vi "make_gasid_unit_ring.vi"() -> ()   [LabVIEW 2013]
uses:
  <vilib>/Utility/file.llb/Read From Spreadsheet File (string).vi
panel:
  in  "uom1":T1(ring)
  in  "gid2":T2(ring)
  out "Duplicates":string[](array[string])
  out "Uniques":string[](array[string])
  out "all rows":string[][](array[string])
  in  "Ring":u16(ring) items=["ERR", "SCCM", "SLM", "%", "V", "MV", "CNT", "NLM", "SLS", "NLS", "SLH", "NLH", "SMLM", "NMLM", "SMLS", "NMLS", "SMLH", "NMLH", "NCCM", "SCCS", "NCCS", "SCCH", "NCCH", "SCFM", "NCFM", "SCFS", "NCFS", "SCFH", "NCFH", "SCMM", "NCMM", "SCMS", "NCMS", "SCMH", "NCMH", "SCIM", "NCIM", "SCIS", "NCIS", "SCIH", "NCIH", "LBM", "LBS", "LBH", "KgM", "KgS", "KgH", "GRM", "GMS", "GRH", "MolM", "MolS", "MolH", "KMolM", "KMolS", "KMolH", "W", "BPS", "Sec", "Min", "Hrs", "WH", "Torr", "Bar", "Pa", "inH2O", "PSIA", "PSIG"]
  in  "file path (dialog if empty)":path
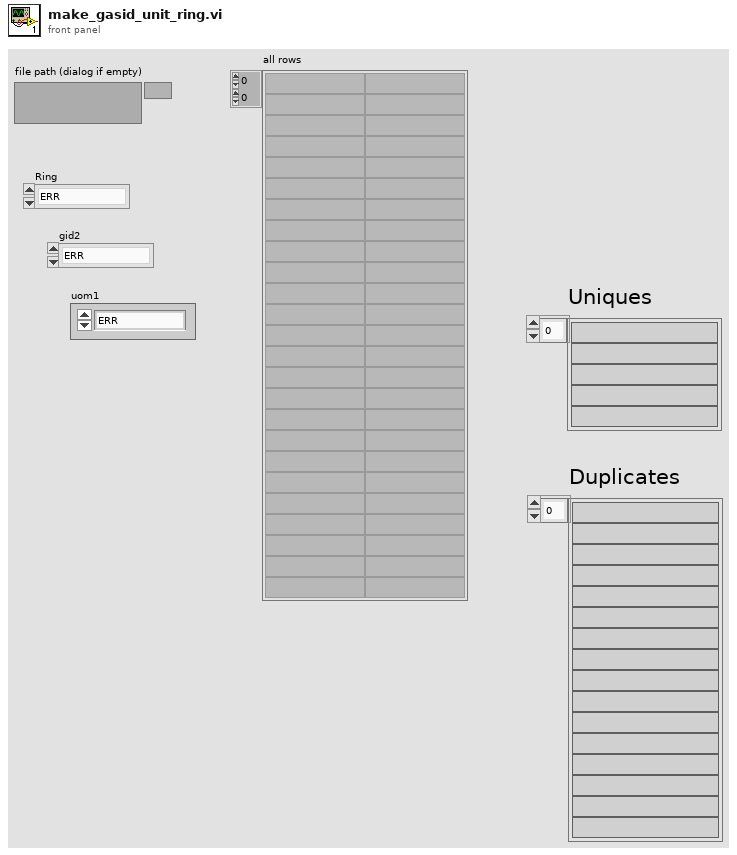
[diagram p1: front panel]
types:
  T1 = enum16{"ERR", "SCCM", "SLM", "%", "V", "MV", "CNT", "NLM", "SLS", "NLS", "SLH", "NLH", "SMLM", "NMLM", "SMLS", "NMLS", "SMLH", "NMLH", "NCCM", "SCCS", "NCCS", "SCCH", "NCCH", "SCFM", "NCFM", "SCFS", "NCFS", "SCFH", "NCFH", "SCMM", "NCMM", "SCMS", "NCMS", "SCMH", "NCMH", "SCIM", "NCIM", "SCIS", "NCIS", "SCIH", "NCIH", "LBM", "LBS", "LBH", "KgM", "KgS", "KgH", "GRM", "GMS", "GRH", "MolM", "MolS", "MolH", "KMolM", "KMolS", "KMolH", "W", "BPS", "Sec", "Min", "Hrs", "WH", "Torr", "Bar", "Pa", "inH2O", "PSIA", "PSIG"}
  T2 = enum16{"ERR", "1", "2", "C3H6O_1", "C2H3N", "C2H2", "Air", "C3H4_1", "NH3", "Ar", "AsH3", "C6H6", "BCl3", "BF3", "Br2", "15", "16", "CBrF3", "C4H10_1", "19", "C4H8_1", "CO2", "CS2", "CO", "CCl4", "COS", "Cl2", "ClF3", "28", "29", "CHCl3", "31", "32", "C4H8_2", "C2N2", "ClCN", "C4H8_3", "C3H6", "H22", "B2H6", "40", "R21", "42", "43", "44", "45", "46", "47", "48", "C2H7N_1", "C2H6O_1", "C2H6S_1", "C4H6_1", "C2H6", "54", "55", "C2H6O_2", "C4H6_2", "C2H7N_2", "C8H10", "60", "61", "C2H5F", "C2H4", "64", "65", "C2H4O", "C2H4N", "68", "C2H6S_2", "F2", "CH2O", "CCl3F", "73", "CClF3", "CF4", "76", "CHF3", "78", "C4H4O", "He", "C3HF7", "HMDS", "83", "C6H14", "C6F6", "C6H12_1", "N2H4", "H2", "HBr", "HCl", "CHN", "HF", "HI", "H2Se", "H2S", "C4H10_2", "97", "C4H8_4", "C5H12_1", "C3H8O_1", "101", "C2H2O", "Kr", "CH4", "CH4O", "106", "C3H4_2", "CH5N", "CH3Br", "CH3Cl", "C7H14", "C3H9N", "C3H8O_2", "C3H8S", "CH3F", "116", "CH3I", "CH4S", "C6H12_2", "C3H6O_2", "Ne", "NO", "N2", "NO2", "N2O4", "NF3", "127", "NOCl", "N2O", "C5H12_2", "C8H18", "O2", "F2O", "O3", "B5H9", ""}
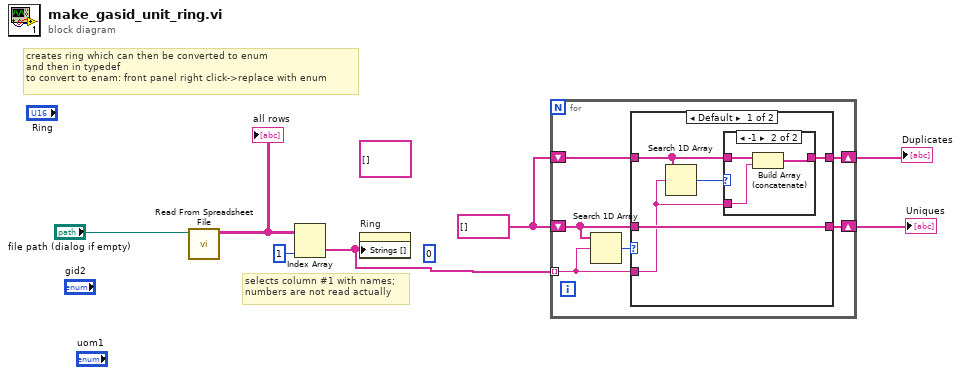
[diagram p0: block diagram]
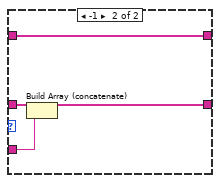
[diagram p3: hidden frame]
diagram:
  w3 = string[] []
  (unwired) 0
  (unwired) string[][] [] ("Array")
  # "selects column #1 with names;\nnumbers are not read actually"
  # "creates ring which can then be converted to enum\nand then in typedef\nto convert to enam: front panel right click->replace with enum"
  n1 = call-poly <vilib>:"Read From Spreadsheet File.vi"("file path (dialog if empty)"="file path (dialog if empty)") -> ("all rows"=w5:string[][])  [unwired: 6 in, 4 out]
  "all rows" <- w5
  n2 = Index Array(array=w5, index (col)=1 ("disabled index (col)")) -> (element=w1:string[])  [unwired: 1 in]
  n3 = property on="Ring" class="Ring (strict)"("Strings []"=w1) -> ()  [unwired: 2 in, 2 out]
  n4 = for {
    tunnel: w1 -> [w12] mode=indexing
    shift-right: [w11] -> w4
    shift-left: w3 -> [w10]
    shift-right: [w8] -> w2
    shift-left: w3 -> [w9]
    n5 = Search 1D Array(1D array=w10, element=w12) -> (index of element=w13:i32)  [unwired: 1 in]
    n6 = case shown="Default" w13 {
      tunnel: w12 -> [w14 w26]
      tunnel: [w18 w24] -> w11
      tunnel: w10 -> [w18 w25]
      tunnel: w9 -> [w15 w23]
      tunnel: [w17 w23] -> w8
      frame Default {
        n7 = Search 1D Array(1D array=w15, element=w14) -> (index of element=w16:i32)  [unwired: 1 in]
        n8 = case shown="-1" w16 {
          tunnel: [w19 w21] -> w17
          tunnel: w15 -> [w19 w22]
          tunnel: w14 -> [_ w20]
          frame Default {
          }
          frame -1 {
            n9 = Build Array (concatenate)(w22, w20) -> (w21:string[])
          }
        }
      }
      frame -1 {
        n10 = Build Array (concatenate)(w25, w26) -> (w24:string[])
      }
    }
  }
  "Uniques" <- w4
  "Duplicates" <- w2
